vi "observacao_0MQ.vi"() -> ()   [LabVIEW 2012, in "Shared_160.lvlib"]
uses:
  Shared_160.lvlib
  Control 1.ctl
  System.Windows.Forms
  Global_Telescopio.vi
  Global Tabs.vi
panel:
  out "angCup":string caption="DOME Pos"
  out "TargetCup":string caption="DOME Tar"
  out "domeRisc":bool
  out "element":string
  out "size(s)":i32
  out "timeStatShutterAlert":i32
  out "sendCommandShutter":bool
  out "shutterTimeOld":i32
  out "LEAF":i32
  in  "Default":string="DEFAULT"
  out "Flag ativo DEC":bool
  out "Flag ativo AH":bool
  out "Flag de erro p/ apagar lampada":bool
  out "Cont-ShutOpen":timestamp
  out "Flag-ShutClose":bool
  out "Flag-ShutOpen":bool
  in  "erro lig":i32=3
  in  "erro des":i32=3
  in  "xxz":string
  out "Flag desligar":bool
  out "Flag ligar":bool
  out "Flag Stop":bool
  in  "AUX LAMPADA":bool
  out "Apontou":bool caption="Working Area"
  in  "AUX ABA":bool
  out "error out 5":errorcluster
  in  "error in (no error)":errorcluster
  out "AH_Destino":dbl format="%.9g"
  out "CONT DEC UTILS":i32
  out "CR DEC UTILS":i32
  out "CONT AH UTILS":i32
  out "CR AH UTILS":i32
  out "Erro PROTEC":i32=5
  out "Erro Lim":i32=5
  out "Flag Alarm":bool
  out "alarm Time":timestamp
  out "error out 4":errorcluster
  in  "Case Constant\n(See Context Help) 19":bool=TRUE
  in  "Case Constant\n(See Context Help) 18":bool
  in  "Case Constant\n(See Context Help) 17":bool=TRUE
  in  "Case Constant\n(See Context Help) 16":bool
  in  "LedPointing":bool=TRUE
  in  "Case Ct":bool=TRUE
  in  "Case Constant\n(See Context Help) 12":bool=TRUE
  in  "Case Constant\n(See Context Help) 11":bool
  in  "Case Constant\n(See Context Help) 10":bool
  in  "Case Constant\n(See Context Help) 9":bool
  in  "Disabled":u8=2
  in  "Case Constant\n(See Context Help) 8":bool=TRUE
  in  "Case Constant\n(See Context Help) 7":bool=TRUE
  in  "Case Constant\n(See Context Help) 6":bool
  in  "Case Constant\n(See Context Help) 5":bool
  in  "TRUE=HORA\nFALSE=GRAU":bool=TRUE
  in  "Case Constant\n(See Context Help) 4":bool
  in  "Case Constant\n(See Context Help) 3":bool
  in  "Case Constant\n(See Context Help) 2":bool
  in  "Case Constant\n(See Context Help)":bool
  out "TA3":u32
  out "TA2":u32
  out "TF2":u32
  out "TF1":u32
  out "TA1":u32
  out "Tick Cupula":u32
  out "T2 3":u32
  in  "ESTADO ABRIR":string
  in  "ESTADO FECHAR":string
  out "T2 2":u32
  out "T1 2":u32
  out "T2":u32
  out "T1":u32
  out "DEC":string="00 00 00,00"
  out "Hour Angle 2":string="00 00 0,00" caption="AH"
  in  "TIMER TICK":u32
  in  "STOP":bool
  in  "News":bool
  out "AtmosferaStr":string
  in  "BtShutterClose":bool caption="DOME SHUTTER"
  out "HA obs":dbl
  out "Time to Limit":string
  in  "Clear All Messages":bool
  out "FiltroDuplo":bool
  out "ObjCentrado":bool
  out "Timeout PROT":u32
  out "LIMITE":bool
  in  "DestCUP":i16
  in  "DestAH":dbl
  in  "DestDEC":dbl
  in  "M_CUP":i32
  out "TimeoutCUP 2":u32
  out "TimeoutAH 2":u32
  out "TimeoutDEC 2":u32
  in  "Max":dbl=2300.0
  in  "Min":dbl=200.0
  out "error out":errorcluster
  out "TUBO_STAT":string
  out "CUP_STAT":string
  out "DEC_STAT":string
  out "AH_STAT":string
  out "FOCO_ENC":string
  out "DEC_ENC":string
  out "AH_ENC":string
  out "RA on Target":bool
  in  "BtOnTatget":bool
  out "Offset DEC":dbl format="%#.2f"
  out "Offset RA":dbl format="%#.2f"
  out "Mount Fine Movement":bool
  out "Mount Gross Movement":bool
  in  "follow redirects (T)":bool=TRUE
  out "header":string
  out "subarray":string[][](array[string])
  out "Draw Area 4":cluster{"Width":u32, "Height":u32}
  out "Draw Area 3":cluster{"Width":u32, "Height":u32}
  in  "sair":bool
  out "Saida Path string":string
  out "AUX EDITA RA":string caption="Name"
  out "Sideral time":string caption="ST"
  out "UT":string
  out "FLAG SET COORD":bool
  out "AUX EDITA PMDEC":string caption="Name"
  out "AUX EDITA PMRA":string caption="Name"
  out "AUX EDITA EPOCH":string caption="Name"
  out "AUX EDITA DEC":string caption="Name"
  out "AUX EDITA Name":string caption="Name"
  out "Hour Angle":string="00 00 0,00"
  in  "DECTARGET":string
  in  "AHTARGET":string
  out "Zenital angle":dbl
  out "SlideEnviromental":dbl(slide) caption="Progress ..." scale=0.0..100.0
  out "RA AUX":string
  out "EPOCH AUX":string
  out "Draw Area 2":cluster{"Width":u32, "Height":u32}
  out "SYSTEM MESSAGES":string
  out "Data Acquisition Activity":bool
  out "Auto guider Activity":bool
  out "Security Zone":bool
  out "Precess Data out-of-date":bool
  out "D...":bool
  out "C...":bool
  out "B...":bool
  out "A...":bool
  out "DEC on Target":bool
  out "Dome on Target":bool
  out "Remote User in Control":bool
  out "Air Mass":dbl
  out "Epoch":dbl
  out "Right Ascention":string="00 00 00,00"
  out "Declination":string="00 00 00,00"
  out "Azimuth":dbl
  out "Wind Chill":dbl
  out "Boolean 11":bool
  out "Wind Dir":string
  in  "Int/Ext":bool=TRUE
  out "Temperature":dbl
  out "Humidity":dbl
  out "Dew Point":dbl
  out "Wind Speed":dbl
  out "Pressure":dbl
  in  "RESTART METEOR":bool
  in  "VARIABLE \nTRACKING":bool
  out "LED VAR TRACKING":bool
  out "LED GUIDER":bool
  out "Led Chave Dome":bool
  out "LED MOUNT":bool
  in  "GUIDER":bool
  in  "DOME":bool
  in  "MOUNT":bool
  out "NAME":string
  out "DEC":string
  out "RA":string
  in  "Tab Control":T1(tab)=enum."Test Only"
  in  "IMAGE 5":bool
  out "Image":picture
  in  "PictureBox":refnum<k24>(container)
  out "Image 2":picture
  in  "IMAGE 2":bool
  out "error out 3":errorcluster
  out "error out 2":errorcluster
  in  "IMAGE 4":bool
  out "Image 4":picture
  out "pressão atm":string
  out "hum local":string
  out "Temp amb":string
  in  "IMAGE 3":bool
  out "Image 3":picture
  in  "IMAGE 6":bool
  out "Image 3a":picture
  out "C. AH":i32
  out "DOMO_ENC":string
  out "Proteção":bool
  in  "M_PROT":i32
  out "dt":u32
  out "TUBO":bool[](array[boolean])
  out "CUP":bool[](array[boolean])
  out "DEC":bool[](array[boolean])
  out "RA":bool[](array[boolean])
  in  "statCUP":i32
  in  "statAH":i32
  in  "statDEC":i32
  out "statCUP 2":i32
  out "TimeoutCUP":u32
  out "Azimute cup":u16
  out "PosCUP":i16
  out "dtAUX2":u32
  out "dtAUX3":u32
  out "PosAH":dbl
  out "PosDEC":dbl
  out "dec=":bool
  out "ah=":bool
  in  "CR AH":i32
  in  "CR DEC":i32
  out "C. DEC":i32
  in  "M_AH":i32
  in  "M_DEC":i32
  in  "Stop All":bool
  in  "Setup, Pointing & Guiding":T2(tab)=enum."POINTING"
  in  "RA Max 2":i32 min=-6 max=23
  in  "RA Min 2":i32 min=-6 max=23
  out "Erro":bool
  in  "MAG Max":dbl min=-9.0 max=100.0
  in  "MAG Min":dbl min=-9.0 max=25.0
  in  "DEC Max":i32 min=-90 max=90
  in  "DEC Min":i32 min=-90 max=90
  in  "RA Max":i32 caption="AH Max" min=-6 max=23
  in  "RA Min":i32 caption="AH Min" min=-6 max=23
  in  "Filter RA":bool
  in  "Slide old":i32
  out "Tot Linhas":i32
  in  "Open BSC":bool
  in  "Slide":dbl(slide) min=0.0 max=24.0 step=0.024 scale format="%#_3g"
  in  "EDIT":bool
  in  "Insert":bool
  out "List File":string
  in  "Upload":bool
  in  "Open":bool
  in  "Save AS":bool
  in  "Save":bool
  in  "Clear ALL":bool
  in  "SET coord":bool
  in  "Delete":bool
  in  "Multicolumn Listbox":i32[](listbox)
  out "ScaleMin":string
  out "ScaleMax":string
  out "DEC obs":dbl format="%.9f"
  out "RA obs":dbl format="%.9f"
  in  "ChkPointPrecessed":bool
  in  "Processa Centragem":bool
  out "PM_DEC":string
  out "PM_RA":string
  out "LedPointing":bool caption="Telescope Pointing"
  out "TimeoutAH":u32
  out "TimeoutDEC":u32
  out "AtualDEC":dbl format="%.9f"
  out "MeanDEC":string
  out "MeanRA":string
  in  "MAG":string
  out "Zenital Angle":string
  out "Air Mass":string
  out "Tempo Obs":string
  in  "BtPointPrecess":bool
  in  "ChkCalGlobal":bool=TRUE
  in  "ChkCalLocal":bool caption="Use Local Zero"
  in  "ChkPoinLampOFF":bool=TRUE
  in  "ChkPointRNA":bool
  in  "ChkModel":bool=TRUE
  in  "ChkWindDown":bool
  in  "ChkOpenShutter":bool
  in  "ChkDomeEnable":bool
  out "LedPointWorkArea":bool caption="Working Area"
  in  "BtTargetPoint":bool
  out "StrPointTargetDEC":string caption="Declination"
  out "StrPointTargetRA":string caption="Right Ascension"
  in  "BtPointObjClear":bool
  in  "StrPointObjPMDEC":string caption="DEC Proper Motion"
  in  "StrPointObjPMRA":string caption="RA Proper Motion"
  in  "StrPointObjName":string caption="Name"
  in  "StrPointObjEpoch":string caption="Epoch"
  in  "StrPointObjDEC":string caption="Declination"
  in  "StrPointObjRA":string caption="Right Ascension"
  out "MOV_IDX_DEC":bool
  out "MOV_IDX_AH":bool
  out "LatchDeslocDEC":dbl caption="DEC"
  out "LatchDeslocRA":dbl caption="RA"
  in  "ClearDeslocDEC":bool
  in  "ClearDeslocRA":bool
  out "DeslocDEC":dbl caption="DEC" format="%#.1f"
  out "DeslocRA":dbl caption="RA" format="%#.1f"
  in  "Delete Calagem":bool
  in  "Global":bool caption="Local"
  in  "Calagem":bool
  in  "Up HS":bool
  in  "Right HS":bool
  in  "Down HS":bool
  in  "Left HS":bool
  in  "Velocity (arcsec/sec)":i32(slide) min=0 max=600 scale=0.0..600.0
  in  "BtPrecGO":bool
  in  "BtPrecCentrar":bool
  in  "PreciseOffsetDEC":dbl caption="DEC" min=-10000.0 max=10000.0 step=1.0 format="%.3g"
  in  "PreciseOffsetRA":dbl caption="RA . cos(delta)" min=-10000.0 max=10000.0 step=1.0 format="%.3g"
  in  "Habilita Movimento":bool=TRUE
  in  "Y STAR":i32=1 min=1 max=400 step=1
  in  "X STAR":i32=1 min=1 max=400 step=1
  in  "XY CENTER":bool
  in  "Y CENTER":i32=1 min=1 max=400 step=1
  in  "X CENTER":i32=1 min=1 max=400 step=1
  in  "ClearRA":bool
  in  "ClearDEC":bool
  in  "DEC RATE":i32 min=-2000 max=2000 step=1
  in  "RA  RATE":i32 min=-2000 max=2000 step=1
  in  "focusStop":bool
  out "old":i32 min=0 max=360
  in  "Velocity":dbl(slide)=1.0 caption="(max = 500 u/s)" min=0.1 max=100.0 step=1.0 scale=0.1..100.0
  in  "focusHome":bool
  out "focusStatus":string="            Focus Status"
  out "focuAlarm":bool caption="Motor temp."
  out "focusHoming":bool caption="Homing"
  out "focusMoving":bool caption="Moving"
  out "focusConnected":bool
  out "focusInitialized":bool
  in  "SetDefaultFocus":bool
  out "Foco":dbl(slide) caption="1" scale=0.0..50000.0
  in  "Setpoint":dbl=200.0 caption="Target" min=0.0 max=50700.0 step=1.0
  in  "focusGo":bool
  in  "Focus +":bool caption="Focus Out (+)"
  in  "Focus -":bool caption="Focus In (-)"
  in  "New Angle":string="    0.0"
  out "Default Angle":string="      0.00"
  in  "SetRotatorDefAngle":bool
  in  "Set Rotator Angle":bool
  out "Rotator Angle":string="  0.00" caption="for  GUIDING"
  out "StatShutterFile":string
  out "Command":string
  in  "CCW":bool
  out "RefreshShutterState":bool
  in  "BtParavStop":bool
  in  "BtParavUp":bool
  in  "BtParavDown":bool
  out "LedShutter":bool
  out "TimeoutTrap":u32
  out "StatShutter":string caption="Control State"
  in  "BtShutClose":bool
  in  "BtShutOpen":bool
  out "StatDome":string caption="Control State"
  in  "BtDomeSTOP":bool
  in  "BtDomeGO":bool caption="DOME"
  in  "DomeNewPos":i32=30 caption="New Position" min=1 max=360
  out "AngCup":i16 caption="Position"
  in  "CW":bool
  in  "BtUtilPark":bool
  out "LED ACTION":bool
  out "LED MODE":bool
  in  "ACTION":bool
  in  "MODE":bool
  in  "Default Met":bool=TRUE
  in  "PROTEÇÃO":bool
  in  "STOP":bool
  in  "Enable Centragem":bool=TRUE
  in  "GO":bool
  in  "StrPointObjDEC 2":string caption="DEC"
  in  "StrPointObjRA 2":string caption="AH"
  out "MOVING":bool
  in  "FLAT-FIELD":bool
  in  "ECASS":bool
  in  "BtUtilZenith":bool
  in  "TabInstrumento":T3(tab)=enum."Cam 1"
  out "Posição Rede":i32=10 caption="Largura da Fenda" min=10 max=5000 step=1
  in  "HomePrisma":T4 caption="DOME"
  in  "HomeEspelho":T4 caption="DOME"
  in  "HomeFenda":T4 caption="DOME"
  in  "IronArc":bool=TRUE
  out "Boolean":bool
  out "Largura da Fenda 2":dbl=10.0 caption="Largura da Fenda" min=10.0 max=5000.0 step=1.0
  in  "Prisma das Lâmpadas":bool
  out "Position":string
  in  "Largura da Fenda":dbl=10.0 min=10.0 max=5000.0 step=1.0
  in  "Go Largura da Fenda":bool caption="DOME"
  in  "Angulo da rede de difração":i32=10 caption="Ângulo da Rede" min=10 max=99989 step=1
  in  "Go Angulo de Difração":bool caption="DOME"
  in  "Incand":bool=TRUE
  in  "Neon":bool=TRUE
  in  "Cathode":bool=TRUE
  out "Ang. Fenda":dbl
  in  "Go_Coudé":bool
  in  "Radio Buttons":enum32{"Azul", "Visível", "Vermelho"}(radio)
  out "EndTime":u32
  out "ledAzul":bool
  out "ledVisivel":bool
  out "ledVermelho":bool
  in  "MENSAGEM":string="EM MOVIMENTO"
  out "MENSAGEM 2":string="EM MOVIMENTO"
  out "#2":bool
  out "#3":bool
  out "#4":bool
  out "PosSecundario":bool
  out "Cjto_3":bool
  out "EspAtual":string
  out "parou":bool
  out "parou 2":bool
  out "Posição Espelho":dbl=10.0 caption="Largura da Fenda" min=10.0 max=5000.0 step=1.0
  out "parou 3":bool
  out "Output Message":string
  in  "stopEcass":bool
  out "SlideEcass":u8(slide) caption="Espelho movendo..." max=100 scale=0.0..100.0
  out "LedRep":bool
  out "LedCal":bool
  in  "Sent_EspLampCass":bool
  out "LedHe":bool
  out "LedNe":bool
  in  "He-Ar":bool
  in  "Ne":bool
  in  "stopCam1":bool
  out "SlideCam1":u8(slide) caption="Espelho movendo..." max=100 scale=0.0..100.0
  out "LedRepCam1":bool
  out "LedCalCam1":bool
  in  "Sent_EspDesvFeixe":bool
  in  "Go_filtro":bool
  in  "Filtro":string(combo)
  in  "Mover/Parar":bool
  out "Recuar":bool
  in  "Sentido":bool=TRUE
  in  "Velocidade":bool
  out "Rapido":bool
  out "Lento":bool
  out "Avancar":bool
  out "Comando":string
  in  "Mensage Alarme":string="To light up close the Shutter !"
  out "CoudeSel":bool
  in  "Coude":bool
  in  "BtCalFlatField":bool
  in  "ChkCalLamp4":bool
  in  "ChkCalLamp3":bool
  in  "ChkCalLamp2":bool
  in  "ChkCalLamp1":bool
  in  "BtCalTurnOff":bool
  in  "BtCalTurnOn":bool
  out "StrongSel":bool
  out "MediumSel":bool
  out "WeakSel":bool
  in  "Strong":bool
  in  "Medium":bool
  in  "Weak":bool
  # "TELESCOPE CONTROL SYSTEM\nPICO DOS DIAS OBSERVATORY"
  # "Status Information"
  # "System Positions"
  # "Environmental Status"
  # "(+/-2)"
  # "EXT"
  # "INT"
  # "mBar"
  # "o"
  # "C"
  # "Km/h"
  # "%"
  # "o"
  # "o"
  # "C"
  # "C"
  # "CLOUSURE LIMITS"
  # "Wind Speed            >  70 Km/h\nRelative Humidity    >  97 %\nInternal Dewpoint  <  0.5  C\nExternal Dewpoint <  1.0  C"
  # "OBJECT"
  # "TRACKING ENABLE"
  # "Conector 4"
  # "Conector 3"
  # "ALARME\nATENÇÃO\nERROS\nOCUPADO"
  # "Proteção\n\nTracking\nVar_Track"
  # "LCB\nTRAP\nPARAV"
  # "Rapido\nLigeiro\nFino\nRun"
  # "Rapido\nCW\nCCW\nMoving"
  # "Motor\nIDX_Rdy\nManual"
  # "BSC FILTERS"
  # "LIST FILE"
  # "OBJECT INPUT"
  # "TARGET"
  # "OPTIONS"
  # "MANUAL OFFSET"
  # "PRECISE OFFSET"
  # "N"
  # "E"
  # "W"
  # "arcsec"
  # "arcsec"
  # "S"
  # "DISPLACEMENT"
  # "CALAGEM"
  # "PODE NÃO FUNCIONAR CORRETAMENTE!"
  # "STAR CENTERING"
  # "VAR. TRACKING"
  # "AUTO-GUIDER COORDINATES"
  # "1) Entrar X e Y do cursor do Autoguider correspondente à posição de centragem nas entradas X CENTER e Y CENTER. \n2) Após apontamento, entrar em X STAR e Y STAR os valores de X e Y do Autoguider com o \"Guide Box\" sobre o objeto apontado. \n3) Clicar em MOVE STAR TO CENTER."
  # "(instrument)"
  # "May take many\ntens of seconds"
  # "Continuous Movement"
  # "%"
  # "ATENÇÃO:\nO Rotator ainda não está integrado ao sistema de controle e como sua posição afeta a guiagem, sempre que o rotator for girado manualmente é necessário digitar o valor de sua nova posição no controle \"New Angle\" e pressionar \"SET NEW\".\n\nPressionar \"SET NEW\" ou \"SET DEFAULT\" não gira o rotator!"
  # "ROTATION"
  # "SHUTTER"
  # "WINDSCREEN"
  # "Covers"
  # "FIXED POSITIONS"
  # "Acquisition System\nON TARGET command"
  # "Select one Mirrror"
  # "Mirror #2"
  # "Mirror #3"
  # "Mirrors Drivers"
  # "Lâmpadas de Calibração"
  # "Espelho das Lâmpadas de Calibração"
  # "Posição"
  # "Repouso"
  # "Ativo"
  # "LIGA"
  # "LIGA"
  # "DESL."
  # "DESL."
  # "Espelho do Eucalyptus"
  # "Roda de filtros"
  # "Posição"
  # "Repouso"
  # "Ativo"
  # "Espelho de Campo"
  # "Recuar"
  # "Avançar"
  # "Rápido"
  # "Lento"
  # "CALIBRATION LAMPS"
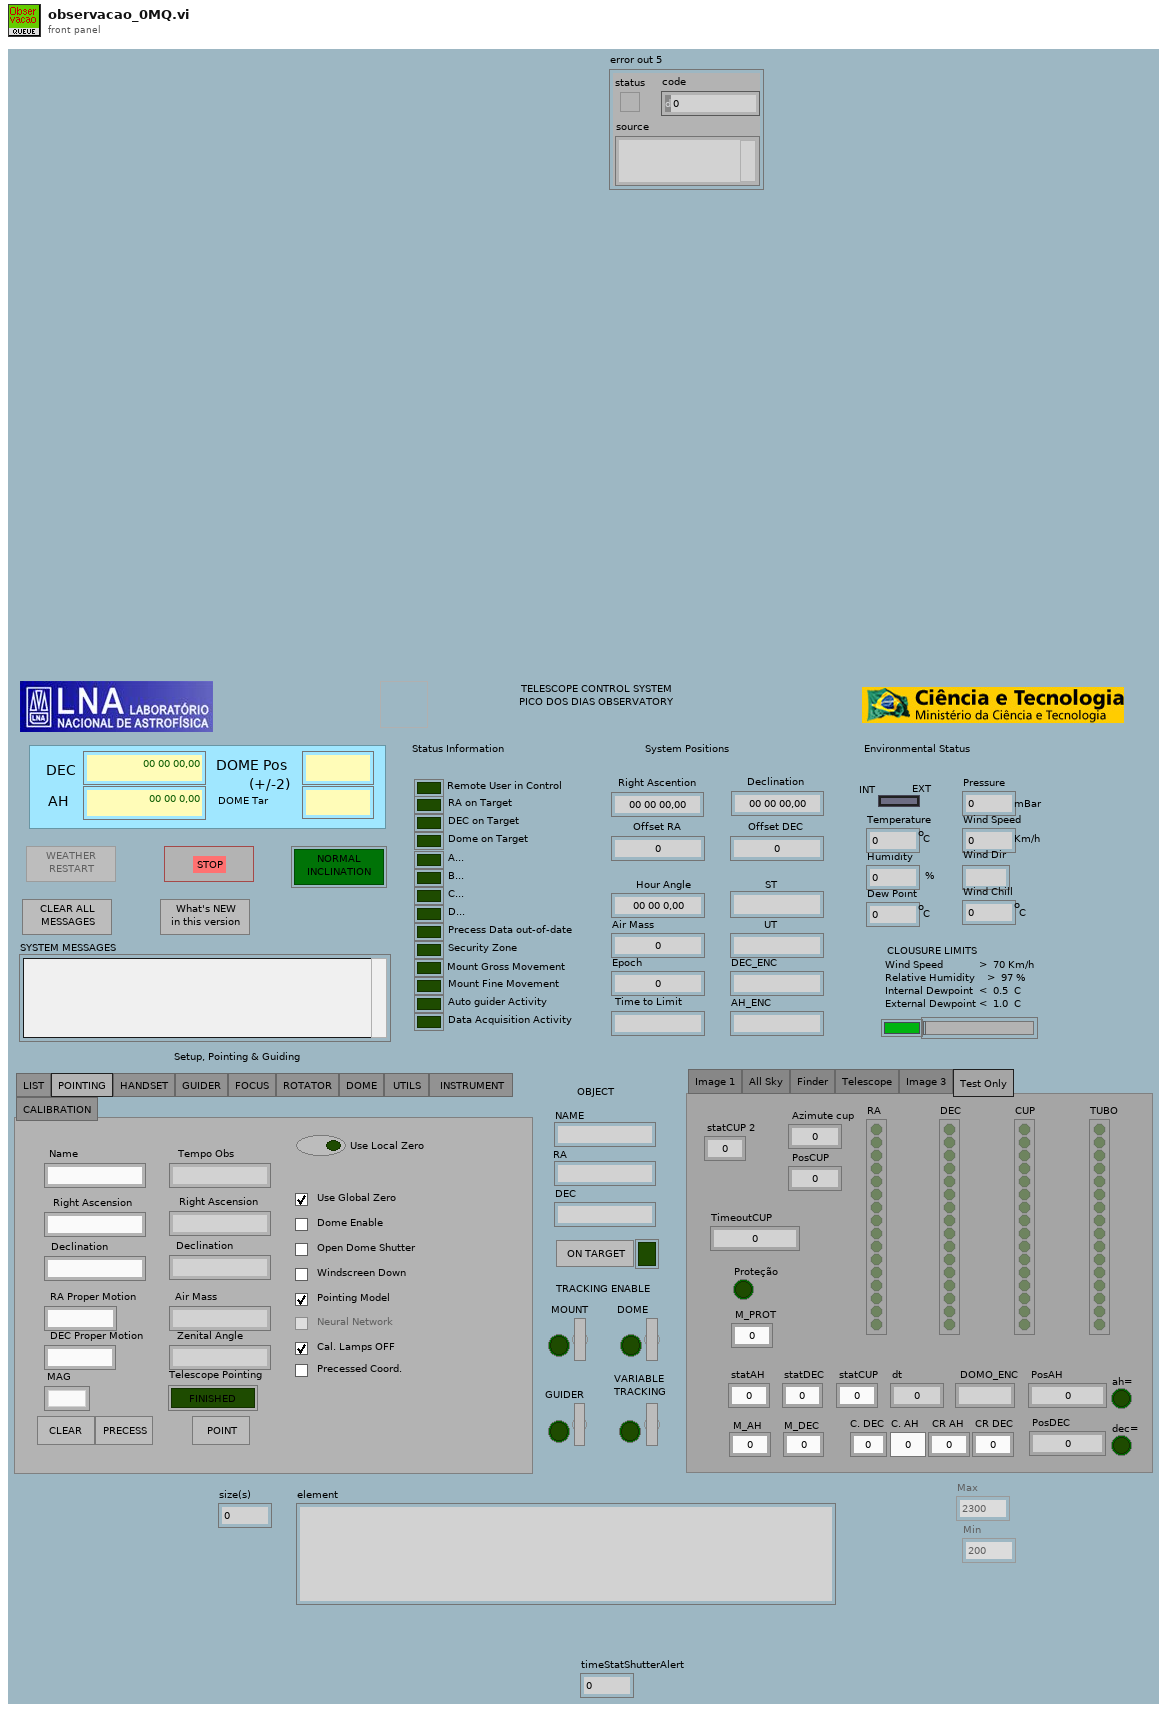
[diagram p1: front panel]
types:
  T1 = enum32{"Image 1", "All Sky", "Finder", "Telescope", "Image 3", "Test Only"}
  T2 = enum32{"LIST", "POINTING", "HANDSET", "GUIDER", "FOCUS", "ROTATOR", "DOME", "UTILS ", " INSTRUMENT ", "CALIBRATION"}
  T3 = enum32{"Coude", "Casseg.", "Eucalyp.", "Cam 1", "Cam 2", "Cam IV.", "Polarim.", "Fotrap"}
  T4 = typedef "Control 1.ctl" = bool
  T5 = enum8{"Enabled", "Disabled", "Disabled and Grayed Out"}
  T6 = enum32{"Page Enabled", "Page Disabled", "Page Disabled & Grayed"}
  T7 = enum16{"open", "replace", "create", "open or create", "replace or create", "replace or create with confirmation"}
  T8 = enum16{"open", "open or create", "create or replace", "create"}
  T9 = enum16{"open", "open or create", "create or replace", "create", "open (read only)"}
  T10 = typedef "LVRemotePanelConnectionsTypeDef.ctl" = cluster{"VI Name":string, "Remote":string, "UserName":string, "Port":i32, "Status":enum32{"Viewing", "Waiting For Control", "Controlling"}, "Create Time":timestamp, "Status Time":timestamp, "Control End Time":timestamp}[]
  T11 = cluster{"absolute":bool, "alarm":bool, "broker":string, "cmd":cluster{"clientId":dbl, "clientTransactionId":dbl, "clientName":string, "action":string}, "connected":bool, "controller":string, "device":string, "error":string, "homing":bool, "initialized":bool, "isMoving":bool, "maxSpeed":dbl, "maxStep":dbl, "position":dbl, "tempComp":bool, "tempCompAvailable":bool, "temperature":dbl, "timestamp":string, "version":string}
  T12 = cluster{"clientId":dbl, "clientTransactionId":dbl, "clientName":string, "action":string}
  T13 = cluster{"left":i16, "top":i16, "right":i16, "bottom":i16}
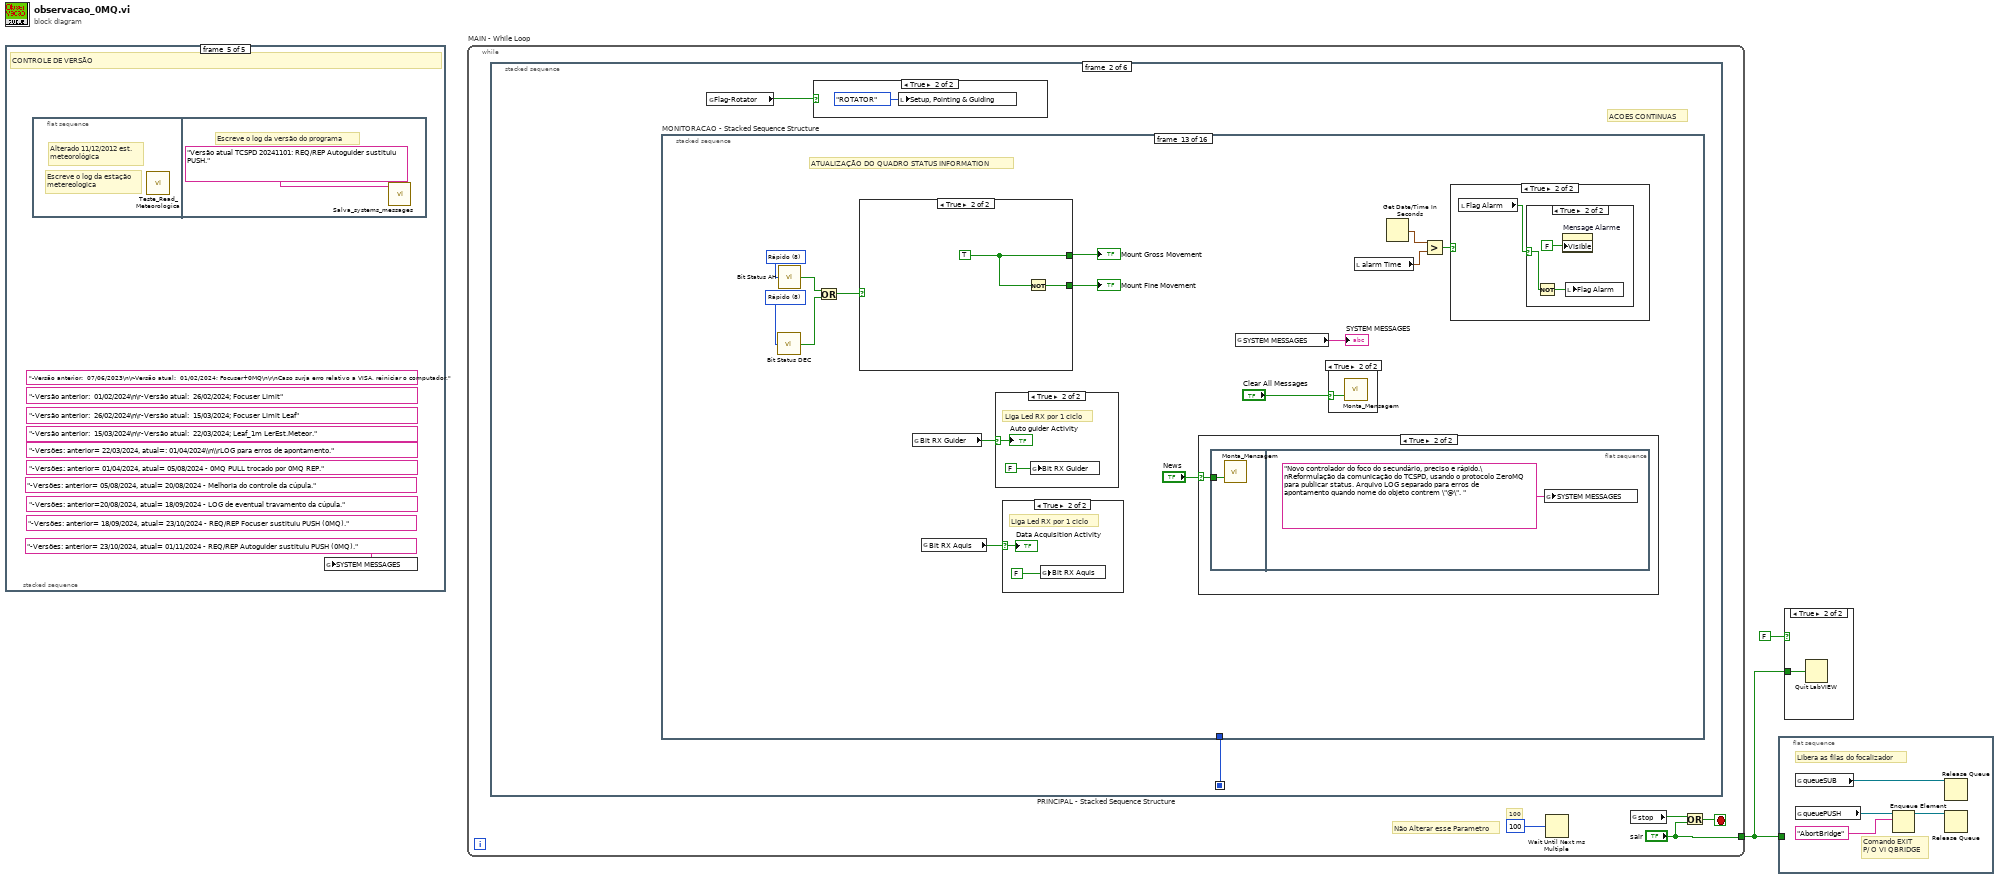
[diagram p0: block diagram]
diagram:
  n1 = stacked-sequence {
    frame #0 {
      w4 = 0 ("estado")
      w3 = ""
      w6 = TRUE ("ChkDomeEnable")
      w5 = FALSE ("Set aux")
      # "RESET DE VARIÁVEIS E CONTROLES"
      n2 = local write "GO"(w5) -> ()
      n3 = local write "MOV_IDX_AH"(w5) -> ()
      n4 = local write "MOV_IDX_DEC"(w5) -> ()
      n5 = local write "Flag ativo AH"(w5) -> ()
      n6 = local write "FLAG SET COORD"(w5) -> ()
      n7 = local write "MOVING"(w5) -> ()
      n8 = local write "Flag ativo DEC"(w5) -> ()
      n9 = local write "DEC on Target"(w5) -> ()
      n10 = local write "RA on Target"(w5) -> ()
      n11 = local write "Erro"(w5) -> ()
      n12 = local write "ChkPointPrecessed"(w5) -> ()
      n13 = local write "ChkOpenShutter"(w5) -> ()
      n14 = local write "Enable Centragem"(w5) -> ()
      n15 = local write "Cathode"(w5) -> ()
      n16 = local write "Neon"(w5) -> ()
      n17 = local write "Incand"(w5) -> ()
      n18 = local write "Dome on Target"(w5) -> ()
      n19 = local write "LedShutter"(w5) -> ()
      n20 = local write "MOUNT"(w5) -> ()
      n21 = local write "Apontou"(w5) -> ()
      n22 = local write "Precess Data out-of-date"(w5) -> ()
      n23 = local write "Flag Stop"(w5) -> ()
      n24 = local write "Flag-ShutOpen"(w5) -> ()
      n25 = local write "MODE"(w5) -> ()
      n26 = local write "ACTION"(w5) -> ()
      n27 = local write "LED ACTION"(w5) -> ()
      n28 = local write "Flag-ShutClose"(w5) -> ()
      n29 = local write "LED MODE"(w5) -> ()
      n30 = local write "Flag de erro p/ apagar lampada"(w5) -> ()
      n31 = global write "Global_Telescopio.vi" "Default Met"(w5) -> ()
      n32 = global write "Global_Telescopio.vi" "Flag-Rotator"(w5) -> ()
      n33 = global write "Global_Telescopio.vi" "Centragem Via Aquisicao"(w5) -> ()
      n34 = global write "Global_Telescopio.vi" "Botão GO = STOP"(w5) -> ()
      n35 = global write "Global_Telescopio.vi" "AQ Offset Mov"(w5) -> ()
      n36 = global write "Global_Telescopio.vi" "STOP ALL"(w5) -> ()
      n37 = global write "Global_Telescopio.vi" "Bit RX Aquis"(w5) -> ()
      n38 = global write "Global_Telescopio.vi" "Bit RX Guider"(w5) -> ()
      n39 = global write "Global_Telescopio.vi" "Correção Guider"(w5) -> ()
      n40 = global write "Global_Telescopio.vi" "CalGlobal"(w5) -> ()
      n41 = global write "Global_Telescopio.vi" "CalLocal"(w5) -> ()
      n42 = global write "Global_Telescopio.vi" "ObjCentrado"(w5) -> ()
      n43 = global write "Global_Telescopio.vi" "LIMITE"(w5) -> ()
      n44 = local write "ChkDomeEnable"(w6) -> ()
      n45 = local write "RefreshShutterState"(w6) -> ()
      n46 = local write "AUX ABA"(w6) -> ()
      n47 = local write "AUX LAMPADA"(w6) -> ()
      n48 = local write "erro lig"(w4) -> ()
      n49 = local write "erro des"(w4) -> ()
      n50 = local write "statDEC"(w4) -> ()
      n51 = local write "statAH"(w4) -> ()
      n52 = local write "statCUP"(w4) -> ()
      n53 = local write "TIMER TICK"(w4) -> ()
      n54 = local write "Tick Cupula"(w4) -> ()
      n55 = local write "CR AH"(w4) -> ()
      n56 = local write "CR DEC"(w4) -> ()
      n57 = global write "Global_Telescopio.vi" "CupStartPos"(w4) -> ()
      n58 = local write "RA"(w3) -> ()
      n59 = local write "DEC"(w3) -> ()
      n60 = local write "NAME"(w3) -> ()
      n61 = local write "MAG"(w3) -> ()
      n62 = local write "StrPointObjName"(w3) -> ()
      n63 = local write "StrPointObjRA"(w3) -> ()
      n64 = local write "StrPointObjDEC"(w3) -> ()
      n65 = local write "StrPointObjEpoch"(w3) -> ()
      n66 = local write "StrPointObjPMRA"(w3) -> ()
      n67 = local write "StrPointObjPMDEC"(w3) -> ()
      n68 = local write "StrPointTargetRA"(w3) -> ()
      n69 = local write "StrPointTargetDEC"(w3) -> ()
      n70 = local write "AUX EDITA Name"(w3) -> ()
      n71 = local write "AUX EDITA RA"(w3) -> ()
      n72 = local write "AUX EDITA DEC"(w3) -> ()
      n73 = local write "AUX EDITA EPOCH"(w3) -> ()
      n74 = local write "AUX EDITA PMRA"(w3) -> ()
      n75 = local write "AUX EDITA PMDEC"(w3) -> ()
      n76 = local write "Tempo Obs"(w3) -> ()
      n77 = local write "ScaleMax"(w3) -> ()
      n78 = local write "ScaleMin"(w3) -> ()
      n79 = local write "Zenital Angle"(w3) -> ()
      n80 = local write "Air Mass"(w3) -> ()
      n81 = local write "Position"(w3) -> ()
      n82 = local write "angCup"(w3) -> ()
    }
    frame #1 {
      w7 = TRUE ("GUIDING")
      w10 = string[][] [] ("Item Names")
      w12 = T5."Enabled" ("Disabled")
      # "INICIALIZAÇÃO DE PROPRIEDADES"
      n83 = property on="Setup, Pointing & Guiding" class="TabCtl (strict)"() -> ("Pages"=w9:refnum<vi>[])  [unwired: 2 in, 2 out]
      n84 = property on="Setup, Pointing & Guiding" class="TabCtl (strict)"("Page Selector Visible"=TRUE) -> ()  [unwired: 2 in, 2 out]
      n85 = property on="BtPointObjClear" class="Bool"("DisabledEnum"=w12) -> ()  [unwired: 2 in, 2 out]
      n86 = property on="BtPointPrecess" class="Bool"("DisabledEnum"=w12) -> ()  [unwired: 2 in, 2 out]
      n87 = property on="PROTEÇÃO" class="Bool (strict)"("Disabled"=w12) -> ()  [unwired: 2 in, 2 out]
      n88 = property on="FLAT-FIELD" class="Bool (strict)"("Disabled"=w12) -> ()  [unwired: 2 in, 2 out]
      n89 = property on="BtUtilZenith" class="Bool (strict)"("Disabled"=w12) -> ()  [unwired: 2 in, 2 out]
      n90 = property on="ECASS" class="Bool (strict)"("Disabled"=w12) -> ()  [unwired: 2 in, 2 out]
      n91 = property on="BtUtilPark" class="Bool (strict)"("Disabled"=w12) -> ()  [unwired: 2 in, 2 out]
      n92 = property on="ACTION" class="Bool (strict)"("Disabled"=T5."Disabled and Grayed Out") -> ()  [unwired: 2 in, 2 out]
      n93 = property on="Setup, Pointing & Guiding" class="TabCtl (strict)"("MultColors"=TRUE ("Allow Multiple Colors")) -> ()  [unwired: 2 in, 2 out]
      n94 = property on="LedPointWorkArea" class="Bool (strict)"("Visible"=TRUE ("GUIDING")) -> ()  [unwired: 2 in, 2 out]
      n95 = property on="Mensage Alarme" class="Str"("Visible"=FALSE, "Blinking"=TRUE) -> ()  [unwired: 2 in, 2 out]
      n96 = property on="LedPointing" class="Bool (strict)"("Visible"=FALSE ("Set aux")) -> ()  [unwired: 2 in, 2 out]
      n97 = for {
        tunnel: w9 -> [w24] mode=indexing
        # "HABILITA TODAS AS ABAS"
        n98 = property class="Page"(reference=w24, "Page Enabled State"=T6."Page Enabled") -> ()  [unwired: 1 in, 2 out]
      }
      n99 = control-ref of="BtTargetPoint"() -> (w15:refnum<vi>)
      n100 = control-ref of="Erro"() -> (w17:refnum<vi>)
      n101 = property on="domeRisc" class="Bool"("Visible"=FALSE ("Set aux")) -> ()  [unwired: 2 in, 2 out]
      n102 = property on="domeRisc" class="Bool"("Blinking"=w7) -> ()  [unwired: 2 in, 2 out]
      n103 = property class="Bool (strict)"(reference=w17, "Boolean Text.Text"="") -> ()  [unwired: 1 in, 2 out]
      n104 = property class="Bool"(reference=w15, "Boolean Text.Text"="POINT") -> ()  [unwired: 1 in, 2 out]
      n105 = property on="Multicolumn Listbox" class="MCListbox (strict)"("Item Names"=w10) -> ()  [unwired: 2 in, 2 out]
      n106 = local write "subarray"(w10) -> ()
      "domeRisc" <- w7
    }
    frame #2 {
      w26 = "REPOUSO" ("y")
      # "MUDANÇA 22/6/11:\nÂngulo do rotator muda ao reiniciar o PC."
      # "Iinicializando o timer do shutter"
      # "INICIALIZAÇÃO DE CONTROLES"
      n107 = Get Date/Time In Seconds() -> (seconds since 1Jan1904=→"alarm Time":timestamp)
      n108 = local write "Default Met"(TRUE ("Default Met")) -> ()
      n109 = global read "Global_Telescopio.vi" "rotator_def"() -> (w25:string)
      n110 = global read "Global_Telescopio.vi" "Instrum"() -> (w30:u16)
      n111 = local write "Multicolumn Listbox"(i32[] [0] ("Multicolumn Listbox")) -> ()
      n112 = local write "ESTADO FECHAR"(w26) -> ()
      n113 = local write "TabInstrumento"(w30) -> ()
      n114 = property on="TabInstrumento" class="TabCtl (strict)"("Disabled"=u8 0) -> ()  [unwired: 2 in, 2 out]
      n115 = local write "ESTADO ABRIR"(w26) -> ()
      n116 = local write "Rotator Angle"(w25) -> ()
      n117 = local write "Default Angle"(w25) -> ()
      n118 = global write "Global_Telescopio.vi" "guide_ang"(w25) -> ()
      n119 = local write "StatDome"("Stopped" ("Status")) -> ()
      n120 = local write "xxz"("inicio") -> ()
      "Flag Alarm" <- FALSE ("Visible")
      "shutterTimeOld" <- 0 ("shutterTimeOld")
      "sendCommandShutter" <- FALSE ("writeShutterLog")
      "timeStatShutterAlert" <- 0 ("timeStatShutterAlert")
    }
    frame #3 {
      w42 = u16 4 items=["ZERO", "AH", "DEC", "TUBO", "CUP"] ("Controlador")
      w41 = u16 3 items=["ZERO", "AH", "DEC", "TUBO", "CUP"] ("Controlador")
      w39 = u16 2 items=["ZERO", "AH", "DEC", "TUBO", "CUP"] ("Controlador")
      w43 = "PROG" ("Comando")
      w44 = "RESET" ("Comando")
      w38 = u16 1 items=["ZERO", "AH", "DEC", "TUBO", "CUP"] ("Controlador")
      # "0- Alarme\n1-Atenção\n2-Erro\n3-Ocupado\n******************\n4-Proteção\n5-Embreagem\n6-Tracking\n7-Var.Track\n8-Rápido\n9-Ligeiro\n10-Médio\n11-Lento\n12-Em movimento\n13-TBD\n14-TBF\n15-TBF\n16-TBF"
      # "RESET DOS CONTROLADORES E INICIALIZAÇÃO DAS FILAS DO FOCALIZADOR"
      n121 = disable-structure shown="Enabled" {
        frame Disabled {
          w45 = u8 0 ("Disabled")
          w47 = u8 1 ("OutOfRngActMin")
          w49 = FALSE ("Set aux")
          # "ZeroMQ"
          # "iniciação aba focus"
          n122 = stacked-sequence {
            frame #0 {
              n123 = global write "Global Tabs.vi" "Off-foc"(0.0 ("Offset")) -> ()
            }
            frame #1 {
              n124 = call "TX focus FOCO.vi"("Comando"="pos") -> ("pos (deg)"=w53:dbl)  [unwired: 12 in, 2 out]
              n125 = global write "Global_Telescopio.vi" "Foco"(w53) -> ()
              n126 = local write "Foco"(w53) -> ()
              n127 = local write "Setpoint"(w53) -> ()
            }
          }
          n128 = property on="Foco" class="Slide (strict)"("Scale.Range:Minimum"="Min", "Scale.Range:Maximum"="Max") -> ()  [unwired: 2 in, 2 out]
          n129 = property on="Setpoint" class="DigNum (strict)"("Data Entry Limits:Minimum"="Min", "Data Entry Limits:Maximum"="Max", "Response to Value Outside Limits:Maximum"=w47, "Response to Value Outside Limits:Minimum"=w47) -> ()  [unwired: 2 in, 2 out]
          n130 = control-ref of="focusGo"() -> (w51:refnum<vi>)
          n131 = property class="Bool"(reference=w51, "Boolean Text.Text"="GO") -> ()  [unwired: 1 in, 2 out]
          n132 = local write "Focus +"(w49) -> ()
          n133 = local write "Focus -"(w49) -> ()
          n134 = property on="Focus -" class="Bool (strict)"("Disabled"=w45) -> ()  [unwired: 2 in, 2 out]
          n135 = property on="Focus +" class="Bool (strict)"("Disabled"=w45) -> ()  [unwired: 2 in, 2 out]
          n136 = property on="Setpoint" class="DigNum (strict)"("Disabled"=w45) -> ()  [unwired: 2 in, 2 out]
        }
        frame Enabled {
          w55 = u8 0 ("Disabled")
          w56 = "OFF"
          w60 = "focusQueue" ("string")
          w61 = ""
          # "Inicializa ClientTransactionId"
          # "Cria as filas de comunicação\ncom 0MQ_Bridge_Foco.vi"
          # "ZeroMQ"
          n137 = property on="Focus +" class="Bool (strict)"("BoolText.Text"=w56) -> ()  [unwired: 2 in, 2 out]
          n138 = property on="Focus -" class="Bool (strict)"("BoolText.Text"=w56) -> ()  [unwired: 2 in, 2 out]
          n139 = Concatenate Strings(w60, "PUSH" ("string")) -> (w63:string)
          n140 = Concatenate Strings(w60, "SUB" ("string")) -> (w62:string)
          n141 = global write "Global_Telescopio.vi" "transactionId0MQ"(u64 0 ("transactionId0MQ")) -> ()
          n142 = Obtain Queue(name (unnamed)=w62, element data type=w61) -> (queue out=w59:refnum<queue>)  [unwired: 3 in, 2 out]
          n143 = Obtain Queue(name (unnamed)=w63, element data type=w61) -> (queue out=w58:refnum<queue>)  [unwired: 3 in, 2 out]
          n144 = global write "Global_Telescopio.vi" "queueSUB"(w59) -> ()
          n145 = global write "Global_Telescopio.vi" "queuePUSH"(w58) -> ()
          n146 = property on="Focus -" class="Bool (strict)"("Disabled"=w55) -> ()  [unwired: 2 in, 2 out]
          n147 = property on="Focus +" class="Bool (strict)"("Disabled"=w55) -> ()  [unwired: 2 in, 2 out]
          n148 = property on="Setpoint" class="DigNum (strict)"("Disabled"=w55) -> ()  [unwired: 2 in, 2 out]
        }
      }
      n149 = call "Monta Comando.vi"("Comando"=w44, "Dispositivo"=w43, "Controlador"=w38) -> ()  [unwired: 4 in, 3 out]
      n150 = call "Monta Comando.vi"("Comando"=w44, "Dispositivo"=w43, "Controlador"=w39) -> ()  [unwired: 4 in, 3 out]
      n151 = Wait (ms)(milliseconds to wait=u32 2000) -> ()  [unwired: 1 out]
      n152 = call "Monta Comando.vi"("Comando"=w44, "Dispositivo"=w43, "Controlador"=w41) -> ()  [unwired: 4 in, 3 out]
      n153 = call "Monta Comando.vi"("Comando"=w44, "Dispositivo"=w43, "Controlador"=w42) -> ()  [unwired: 4 in, 3 out]
    }
    frame #4 {
      (unwired) "-Versões: anterior= 18/09/2024, atual= 23/10/2024 - REQ/REP Focuser sustituiu PUSH (0MQ)." ("SYSTEM MESSAGES")
      (unwired) "-Versões: anterior= 05/08/2024, atual= 20/08/2024 - Melhoria do controle da cúpula." ("SYSTEM MESSAGES")
      (unwired) "-Versões: anterior=20/08/2024, atual= 18/09/2024 - LOG de eventual travamento da cúpula." ("SYSTEM MESSAGES")
      (unwired) "-Versões: anterior= 01/04/2024, atual= 05/08/2024 - 0MQ PULL trocado por 0MQ REP." ("SYSTEM MESSAGES")
      (unwired) "-Versões: anterior= 22/03/2024, atual=: 01/04/2024\\n\\rLOG para erros de apontamento." ("SYSTEM MESSAGES")
      (unwired) "-Versão anterior:  26/02/2024\n\r-Versão atual:  15/03/2024; Focuser Limit Leaf" ("SYSTEM MESSAGES")
      (unwired) "-Versão anterior:  01/02/2024\n\r-Versão atual:  26/02/2024; Focuser Limit" ("SYSTEM MESSAGES")
      (unwired) "-Versão anterior:  15/03/2024\n\r-Versão atual:  22/03/2024; Leaf_1m LerEst.Meteor." ("SYSTEM MESSAGES")
      (unwired) "-Versão anterior:  07/06/2023\n\r-Versão atual:  01/02/2024; Focuser+0MQ\n\r\nCaso surja erro relativo a VISA, reiniciar o computador." ("SYSTEM MESSAGES")
      # "CONTROLE DE VERSÃO"
      n154 = flat-sequence {
        frame #0 {
          # "Escreve o log da estação\nmetereologica"
          # "Alterado 11/12/2012 est.\nmeteorológica"
          n155 = call "Teste_Read_Meteorologica.vi"() -> ()  [unwired: 2 in, 1 out]
        }
        frame #1 {
          # "Escreve o log da versão do programa"
          n156 = call "Salva_systems_messages.vi"("Mensagem"="Versão atual TCSPD 20241101: REQ/REP Autoguider sustituiu PUSH." ("message")) -> ()  [unwired: 5 in]
        }
      }
      n157 = global write "Global_Telescopio.vi" "SYSTEM MESSAGES"("-Versões: anterior= 23/10/2024, atual= 01/11/2024 - REQ/REP Autoguider sustituiu PUSH (0MQ)." ("SYSTEM MESSAGES")) -> ()
    }
  }
  n158 = while "MAIN - While Loop" {
    tunnel: ["sair"] -> w1
    stop <- w70 stop-if-true
    # "100"
    # "Não Alterar esse Parametro"
    n159 = stacked-sequence "PRINCIPAL - Stacked Sequence Structure" {
      seq-local: [w75 _ _ _ _ _] -> [_ w78 _ _ _ w4293]
      frame #0 {
        # "CLIENTE REMOTO"
        # "Verifica se Existe Cliente Remoto Conectado"
        n160 = invoke class="VI" method="RP.Client Connections"() -> ("Connections"=w76:T10, "Controller"=w74:i32)  [unwired: 5 in, 3 out]
        n161 = Tick Count (ms)() -> (millisecond timer value=w75:u32)
        n162 = Equal?(x=w74, y=0) -> (x = y?=→"Remote User in Control":bool)
        n163 = global write "Global_Telescopio.vi" "Controller Rem/Loc"(w74) -> ()
        n164 = global write "Global_Telescopio.vi" "Dados do Computador Remoto Conectado"(w76) -> ()
      }
      frame #1 {
        # "ACOES CONTINUAS"
        n165 = stacked-sequence "MONITORACAO - Stacked Sequence Structure" {
          tunnel: w78 -> [_ _ _ w506 _ _ _ _ _ _ _ _ _ _ _ _]
          frame #0 {
            w107 = u16 3 items=["ZERO", "AH", "DEC", "TUBO", "CUP", "CASS", "COUDE"] ("Controlador")
            w115 = u16 4 items=["ZERO", "AH", "DEC", "TUBO", "CUP", "CASS", "COUDE"] ("Controlador")
            w116 = u16 2 items=["ZERO", "AH", "DEC", "TUBO", "CUP", "CASS", "COUDE"] ("Controlador")
            w119 = u16 1 items=["ZERO", "AH", "DEC", "TUBO", "CUP", "CASS", "COUDE"] ("Controlador")
            # "PROCESSO LE ENCODERS"
            # "LEITURA STATUS DOS CONTROLADORES"
            n166 = disable-structure shown="Disabled" {
              frame Disabled {
                # "ZeroMQ"
                # "Grava o valor do foco \natual a cada minuto"
                n167 = Get Date/Time In Seconds() -> (seconds since 1Jan1904=w146:timestamp)
                n168 = Format Date/Time String(time format string (%c)="%S", seconds (now)=w146) -> (date/time string=w145:string)  [unwired: 1 in]
                n169 = Equal?(x=w145, y="00") -> (x = y?=w143:bool)
                n170 = case shown="True" w143 {
                  frame False {
                  }
                  frame True {
                    n171 = local read "Foco"() -> (w150:dbl)
                    n172 = Number To Decimal String(number=w150) -> (decimal integer string=w149:string)  [unwired: 1 in]
                    n173 = call "Log_Foco.vi"("command"=" ", "focValue"=w149, "pathLogFocoString"="C:\\TCS\\LOG\\FOCO\\") -> ()  [unwired: 6 in]
                  }
                }
              }
              frame Enabled {
                # "ZeroMQ"
                n174 = First Call?() -> (First Call?: T/F=w152:bool)
                n175 = case shown="True" w152 {
                  frame False {
                  }
                  frame True {
                    n176 = global read "Global_Telescopio.vi" "transactionId0MQ"() -> (w153:u64)
                    n177 = Increment(x=w153) -> (x+1=w154:u64)
                    n178 = call "Focus PUSH.vi"("action"="STATUS" ("controller"), "clientTransactionId"=w153) -> ()  [unwired: 9 in, 1 out]
                    n179 = global write "Global_Telescopio.vi" "transactionId0MQ"(w154) -> ()
                  }
                }
              }
            }
            n180 = case shown="False" "Case Constant\n(See Context Help)" {
              selector: "Case Constant\n(See Context Help)" -> [_ w269]
              tunnel: [w268 w269] -> w117
              tunnel: w116 -> [w267 _]
              tunnel: [w266 _] -> w118
              tunnel: [w265 _] -> w90
              tunnel: [w264 _] -> w103
              frame False {
                n181 = call "Get Status Controlador.vi"("Controlador"=w267) -> ("Status"=w264:string, "Parametros"=w266:string, "Bits Status"=w265:bool[], "Erro comunicação"=w268:bool)
              }
              frame True {
              }
            }
            "DEC_STAT" <- w103
            "DEC" <- w90
            n182 = case shown="False" "Case Constant\n(See Context Help)" {
              selector: "Case Constant\n(See Context Help)" -> [_ w263]
              tunnel: [w262 w263] -> w114
              tunnel: w115 -> [w261 _]
              tunnel: [w260 _] -> w113
              tunnel: [w259 _] -> w100
              tunnel: [w258 _] -> w102
              frame False {
                n183 = call "Get Status Controlador.vi"("Controlador"=w261) -> ("Status"=w258:string, "Parametros"=w260:string, "Bits Status"=w259:bool[], "Erro comunicação"=w262:bool)
              }
              frame True {
              }
            }
            "CUP_STAT" <- w102
            "CUP" <- w100
            n184 = case shown="False" "Case Constant\n(See Context Help)" {
              selector: "Case Constant\n(See Context Help)" -> [_ w225]
              tunnel: [w224 w225] -> w108
              tunnel: w107 -> [w223 _]
              tunnel: [w222 _] -> w109
              tunnel: [w221 _] -> w98
              tunnel: [w220 _] -> w101
              frame False {
                n185 = call "Get Status Controlador.vi"("Controlador"=w223) -> ("Status"=w220:string, "Parametros"=w222:string, "Bits Status"=w221:bool[], "Erro comunicação"=w224:bool)
              }
              frame True {
              }
            }
            "TUBO_STAT" <- w101
            "TUBO" <- w98
            n186 = case shown="False" "Case Constant\n(See Context Help)" {
              selector: "Case Constant\n(See Context Help)" -> [_ w303]
              tunnel: w119 -> [w302 _]
              tunnel: [w301 _] -> w91
              tunnel: [w300 _] -> w121
              tunnel: [w299 w303] -> w120
              tunnel: [w298 _] -> w104
              frame False {
                n187 = call "Get Status Controlador.vi"("Controlador"=w302) -> ("Status"=w298:string, "Parametros"=w300:string, "Bits Status"=w301:bool[], "Erro comunicação"=w299:bool)
              }
              frame True {
              }
            }
            "AH_STAT" <- w104
            "RA" <- w91
            n188 = call "Testa_Comunicação.vi"("DEC"=w90, "RA"=w91) -> ()  [unwired: 10 in]
            n189 = Index Array(array=w98, index=3) -> (element=w96:bool)
            n190 = case shown="False" w96 {
              tunnel: ["S" "M"] -> w95
              frame False {
              }
              frame True {
              }
            }
            n191 = case shown="False" w120 {
              tunnel: w91 -> [w290 _]
              tunnel: w121 -> [w289 _]
              tunnel: [w287 _] -> w106
              frame False {
                # "Leitura Válida"
                n192 = call <vilib>:"Trim Whitespace.vi"("string"=w289) -> ("trimmed string"=w287:string)  [unwired: 1 in]
                n193 = call "hms_rad.vi"("True = hora"=TRUE, "Texto Graus"=w287) -> ("radianos"=w284:dbl)  [unwired: 3 in]
                n194 = global write "Global_Telescopio.vi" "StatusAH"(w290) -> ()
                n195 = global read "Global_Telescopio.vi" "PosAH"() -> (w286:dbl)
                n196 = Equal?(x=w286, y=w284) -> (x = y?=w285:bool)
                n197 = case shown="False" w285 {
                  tunnel: w284 -> [w293 _]
                  frame False {
                    w292 = 0 ("CR AH")
                    n198 = global write "Global_Telescopio.vi" "PosAH"(w293) -> ()
                    n199 = local write "CR AH"(w292) -> ()
                    n200 = local write "CR AH UTILS"(w292) -> ()
                    "PosAH" <- w293
                    "Flag ativo AH" <- TRUE ("Flag ativo AH")
                  }
                  frame True {
                    n201 = local read "CR AH UTILS"() -> (w295:i32)
                    n202 = local read "CR AH"() -> (w296:i32)
                    n203 = Increment(x=w295) -> (x+1=w294:i32)
                    n204 = Increment(x=w296) -> (x+1=w297:i32)
                    n205 = local write "CR AH UTILS"(w294) -> ()
                    n206 = local write "CR AH"(w297) -> ()
                  }
                }
              }
              frame True {
                # "Erro na Leitura"
              }
            }
            "AH_ENC" <- w106
            n207 = case shown="False" w117 {
              tunnel: w118 -> [w275 _]
              tunnel: w90 -> [w274 _]
              tunnel: [w273 _] -> w105
              frame False {
                # "Leitura Válida"
                n208 = call <vilib>:"Trim Whitespace.vi"("string"=w275) -> ("trimmed string"=w273:string)  [unwired: 1 in]
                n209 = call "hms_rad.vi"("True = hora"=FALSE, "Texto Graus"=w273) -> ("radianos"=w270:dbl)  [unwired: 3 in]
                n210 = global write "Global_Telescopio.vi" "StatusDEC"(w274) -> ()
                n211 = global read "Global_Telescopio.vi" "PosDEC"() -> (w272:dbl)
                n212 = Equal?(x=w272, y=w270) -> (x = y?=w271:bool)
                n213 = case shown="False" w271 {
                  tunnel: w270 -> [w279 _]
                  frame False {
                    w278 = 0 ("CR DEC")
                    n214 = global write "Global_Telescopio.vi" "PosDEC"(w279) -> ()
                    n215 = local write "CR DEC UTILS"(w278) -> ()
                    n216 = local write "CR DEC"(w278) -> ()
                    "PosDEC" <- w279
                    "Flag ativo DEC" <- TRUE ("Flag ativo DEC")
                  }
                  frame True {
                    n217 = local read "CR DEC UTILS"() -> (w281:i32)
                    n218 = local read "CR DEC"() -> (w283:i32)
                    n219 = Increment(x=w281) -> (x+1=w280:i32)
                    n220 = Increment(x=w283) -> (x+1=w282:i32)
                    n221 = local write "CR DEC UTILS"(w280) -> ()
                    n222 = local write "CR DEC"(w282) -> ()
                  }
                }
              }
              frame True {
                # "Erro na Leitura"
              }
            }
            "DEC_ENC" <- w105
            n223 = case shown="False" w114 {
              tunnel: w100 -> [w233 _]
              tunnel: w113 -> [w232 _]
              tunnel: [w231 w256] -> w81
              tunnel: [w230 w257] -> w82
              tunnel: [w228 FALSE] -> w80
              frame False {
                w229 = u16 12 items=["Alarme", "Atencao", "Erro", "Ocupado", "TBD", "LCB", "Trapeira", "Paravento", "DomoRap", "DomoCW", "DomoCCW", "TBD", "Em movimento", "TBD"] ("NomeStatus")
                # "Leitura Válida"
                n224 = global write "Global_Telescopio.vi" "StatusCUP"(w233) -> ()
                n225 = stacked-sequence {
                  tunnel: w232 -> [w239 _ _]
                  tunnel: [w235 _ _] -> w231
                  tunnel: [_ w244 _] -> w230
                  tunnel: [_ _ w246] -> w226
                  tunnel: w229 -> [_ _ w251]
                  tunnel: [w234 _ _] -> w227
                  frame #0 {
                    n226 = call <vilib>:"Trim Whitespace.vi"("string"=w239) -> ("trimmed string"=w235:string)  [unwired: 1 in]
                    n227 = Decimal String To Number(string=w235) -> (number=w238:i32)  [unwired: 2 in, 1 out]
                    n228 = global read "Global_Telescopio.vi" "CupLastEnc"() -> (w237:string)
                    n229 = global write "Global_Telescopio.vi" "PosCUP"(w238) -> ()
                    n230 = Not Equal?(x=w235, y=w237) -> (x != y?=w236:bool)
                    n231 = case shown="True" w236 {
                      tunnel: w235 -> [_ w243]
                      tunnel: [TRUE FALSE] -> w234
                      frame False {
                      }
                      frame True {
                        n232 = call "TickTimeout.vi"() -> ("msTick"=w242:u32)  [unwired: 2 in, 2 out]
                        n233 = global write "Global_Telescopio.vi" "CupLastEnc"(w243) -> ()
                        n234 = global write "Global_Telescopio.vi" "CupTimeLock"(w242) -> ()
                      }
                    }
                  }
                  frame #1 {
                    n235 = global read "Global_Telescopio.vi" "PosCUP"() -> (w245:i16)
                    n236 = call "Checa destino cupula.vi"("Target"=w245) -> ("angCUP"=w244:string)  [unwired: 6 in, 2 out]
                  }
                  frame #2 {
                    n237 = global read "Global_Telescopio.vi" "CupTimeLock"() -> (w250:u32)
                    n238 = call "Bit Status CUP.vi"("NomeStatus"=w251) -> ("StatBit"=w247:bool)
                    n239 = call "TickTimeout.vi"("msInicial"=w250, "msTimeout"=u32 10000) -> ("Timeout"=w248:bool)  [unwired: 2 out]
                    n240 = Select(t=u32 16747264 ("orangeColor"), s=w247, f=u32 16776376 ("yellowColor")) -> (s? t:f=w254:u32)
                    n241 = And(x=w248, y=w247) -> (x .and. y?=w246:bool)
                    n242 = property on="angCup" class="Str"("Text.BGColor"=w254) -> ()  [unwired: 2 in, 2 out]
                  }
                }
                n243 = And(x=w226, y=w227) -> (x .and. y?=w228:bool)
              }
              frame True {
                # "Erro na Leitura"
                n244 = local read "DOMO_ENC"() -> (w256:string)
                n245 = local read "angCup"() -> (w257:string)
              }
            }
            "DOMO_ENC" <- w81
            "angCup" <- w82
            n246 = global write "Global_Telescopio.vi" "MOTOR LIGADO"(w95) -> ()
            n247 = case shown="False" w108 {
              tunnel: w98 -> [w218 _]
              tunnel: w109 -> [w213 _]
              frame False {
                # "Leitura Válida"
                n248 = call <vilib>:"Trim Whitespace.vi"("string"=w213) -> ("trimmed string"=w217:string)  [unwired: 1 in]
                n249 = Decimal String To Number(string=w217) -> (number=w216:i32)  [unwired: 2 in, 1 out]
                n250 = global write "Global_Telescopio.vi" "StatusTUBO"(w218) -> ()
                n251 = global write "Global_Telescopio.vi" "PosFOCO"(w216) -> ()
                n252 = String Subset(string=w213, offset (0)=10, length (rest)=1 ("length (rest)")) -> (substring=→"EspAtual":string)
                n253 = Number To Decimal String(number=w216) -> (decimal integer string=w211:string)  [unwired: 1 in]
                "FOCO_ENC" <- w211
                n254 = Decimal String To Number(string=w211) -> (number=w209:i32)  [unwired: 2 in, 1 out]
                n255 = Greater Than 0?(x=w209) -> (x > 0?=w210:bool)
                n256 = case shown="True" w210 {
                  tunnel: w209 -> [_ w219]
                  frame False {
                  }
                  frame True {
                    n257 = global write "Global_Telescopio.vi" "Foco"(w219) -> ()
                  }
                }
              }
              frame True {
                # "Erro na Leitura"
              }
            }
            n258 = stacked-sequence {
              frame #0 {
                # "Verifica se exite o arquivo da trapeira"
                # "Lê do arquivo qual o estado atual da trapeira"
                n259 = String To Path(string="C:\\TCS\\LOG\\SHUTTER\\SHUTTER.TXT" ("pathLogFocoString")) -> (path=w159:path)
                n260 = call <vilib>:"Check if File or Folder Exists.vi"("path"=w159) -> ("file or folder exists?"=w157:bool, "dup path"=w156:path)  [unwired: 8 in, 1 out]
                n261 = case shown="True" w157 {
                  tunnel: w156 -> [_ w169]
                  frame False {
                    n262 = local write "StatShutterFile"(" " ("StatShutterFile")) -> ()
                  }
                  frame True {
                    n263 = Open/Create/Replace File(file path (use dialog)=w169, operation (0:open)=T7."open", access (0:read/write)=enum16{"read/write", "read-only", "write-only"}."read/write") -> (refnum out=w166:refnum<file>, error out=w161:errorcluster)  [unwired: 3 in, 1 out]
                    n264 = Read from Text File(file (use dialog)=w166, error in=w161) -> (text=w165:string)  [unwired: 2 in, 3 out]
                    n265 = Match Pattern(string=w165, regular expression="SHUTTER") -> (after substring=w163:string)  [unwired: 1 in, 3 out]
                    n266 = call <vilib>:"Trim Whitespace.vi"("string"=w163) -> ("trimmed string"=w162:string)  [unwired: 1 in]
                    n267 = case shown="\"CLOSED\"" w162 {
                      selector: w162 -> [w170 w171]
                      frame "OPENED", Default {
                        "StatShutterFile" <- w170
                      }
                      frame "CLOSED" {
                        n268 = local write "StatShutterFile"(w171) -> ()
                      }
                    }
                  }
                }
              }
              frame #1 {
                n269 = local read "timeStatShutterAlert"() -> (w174:i32)
                n270 = Tick Count (ms)() -> (millisecond timer value=w176:u32)
                n271 = Add(x=w174, y=3000) -> (x+y=w175:i32)
                n272 = Greater Or Equal?(x=w176, y=w175) -> (x >= y?=w172:bool)
                n273 = case shown="True" w172 {
                  frame False {
                  }
                  frame True {
                    n274 = local read "StatShutterFile"() -> (w178:string)
                    n275 = property on="LedShutter" class="Bool (strict)"() -> ("BoolText.Text"=w179:string)  [unwired: 2 in, 2 out]
                    n276 = Not Equal?(x=w179, y=w178) -> (x != y?=w177:bool)
                    n277 = case shown="True" w177 {
                      frame True {
                        n278 = property on="StatShutterFile" class="Str"("Blinking"=TRUE) -> ()  [unwired: 2 in, 2 out]
                      }
                      frame False {
                        n279 = property on="StatShutterFile" class="Str"("Blinking"=FALSE) -> ()  [unwired: 2 in, 2 out]
                      }
                    }
                  }
                }
              }
              frame #2 {
                n280 = disable-structure shown="Disabled" {
                  frame Disabled {
                    n281 = local read "StatShutterFile"() -> (w183:string)
                    n282 = property on="LedShutter" class="Bool (strict)"() -> ("BoolText.Text"=w184:string)  [unwired: 2 in, 2 out]
                    n283 = Not Equal?(x=w184, y=w183) -> (x != y?=w182:bool)
                    n284 = case shown="True" w182 {
                      frame False {
                        n285 = property on="Setup, Pointing & Guiding" class="TabCtl (strict)"() -> ("Pages"=w186:refnum<vi>[])  [unwired: 2 in, 2 out]
                        n286 = Index Array(array=w186, index=6) -> (element=w187:refnum<vi>)
                        n287 = property class="Page"(reference=w187, "FG Color"=u32 12369084) -> ()  [unwired: 1 in, 2 out]
                      }
                      frame True {
                        n288 = property on="Setup, Pointing & Guiding" class="TabCtl (strict)"() -> ("Pages"=w194:refnum<vi>[])  [unwired: 2 in, 2 out]
                        n289 = Index Array(array=w194, index=6) -> (element=w193:refnum<vi>)
                        n290 = property class="Page"(reference=w193) -> ("FG Color"=w190:u32)  [unwired: 1 in, 2 out]
                        n291 = Equal?(x=w190, y=u32 16711680) -> (x = y?=w189:bool)
                        n292 = case shown="True" w189 {
                          frame False {
                            n293 = property on="Setup, Pointing & Guiding" class="TabCtl (strict)"() -> ("Pages"=w196:refnum<vi>[])  [unwired: 2 in, 2 out]
                            n294 = Index Array(array=w196, index=6) -> (element=w197:refnum<vi>)
                            n295 = property class="Page"(reference=w197, "FG Color"=u32 16711680) -> ()  [unwired: 1 in, 2 out]
                          }
                          frame True {
                            n296 = property on="Setup, Pointing & Guiding" class="TabCtl (strict)"() -> ("Pages"=w200:refnum<vi>[])  [unwired: 2 in, 2 out]
                            n297 = Index Array(array=w200, index=6) -> (element=w201:refnum<vi>)
                            n298 = property class="Page"(reference=w201, "FG Color"=u32 12369084) -> ()  [unwired: 1 in, 2 out]
                          }
                        }
                      }
                    }
                  }
                  frame Enabled {
                  }
                }
              }
            }
            n299 = local read "shutterTimeOld"() -> (w89:i32)
            n300 = local read "LedPointing"() -> (w93:bool)
            n301 = local read "MOVING"() -> (w94:bool)
            n302 = local read "sendCommandShutter"() -> (w84:bool)
            n303 = case shown="True" w80 {
